vi "Read name.vi"(8 "error in (no error)":errorcluster, 11 "GuiderName.lvclass in":refnum<class "GuiderName.lvclass">) -> (0 "error out":errorcluster, 2 "guiderName":string, 3 "GuiderName.lvclass out":refnum<class "GuiderName.lvclass">)   [LabVIEW 2014, in "TCSDataDefinitions.lvlib" / "TCSGuiderCommand.lvlib" / "GuiderName.lvclass"]
uses:
  GuiderName.lvclass
  GuiderName.lvclass/GuiderName.ctl
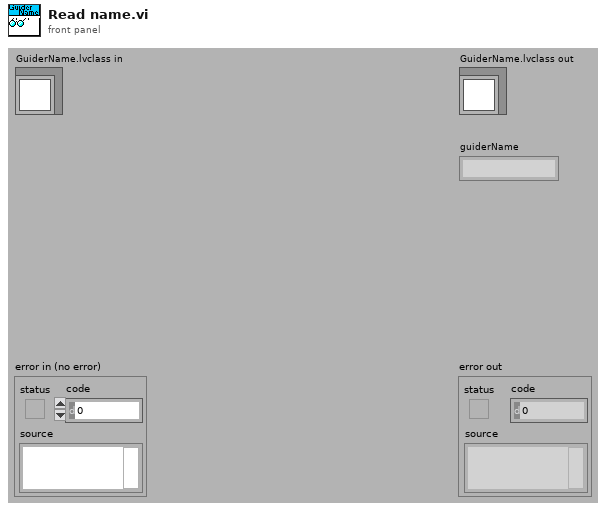
[diagram p1: front panel]
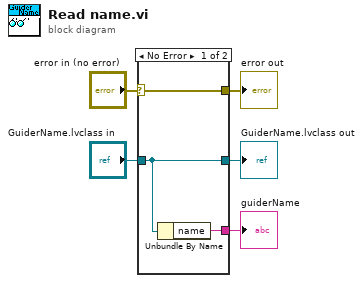
[diagram p0: block diagram]
diagram:
  n1 = case shown="No Error" "error in (no error)" {
    selector: "error in (no error)" -> [w8 w9]
    tunnel: [w8 w9] -> w4
    tunnel: [w7 w10] -> w2
    tunnel: "GuiderName.lvclass in" -> [w7 w10]
    tunnel: [w6 _] -> w1
    frame No Error {
      n2 = Unbundle By Name(w7) -> ("name"=w6:string)
    }
    frame Error {
    }
  }
  "error out" <- w4
  "GuiderName.lvclass out" <- w2
  "guiderName" <- w1
